vi "Init from Time Stamp.vi"(8 "error in":errorcluster, 10 "Time Stamp":timestamp format="%<%x %.3X>T", 11 "Time Stamp in":refnum<class "Time Stamp.lvclass">) -> (0 "error out":errorcluster, 3 "Time Stamp out":refnum<class "Time Stamp.lvclass">)   [LabVIEW 2023, in "HAL.lvlib" / "Time Stamp.lvclass"]
uses:
  Time Stamp.lvclass
  Time Stamp.lvclass/Time Stamp.ctl
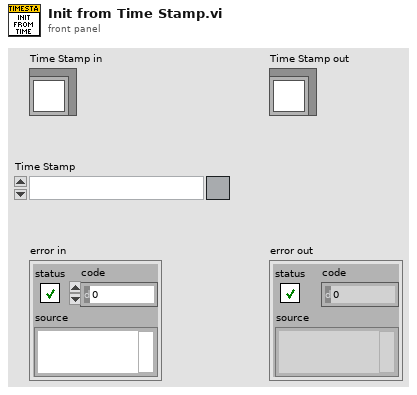
[diagram p1: front panel]
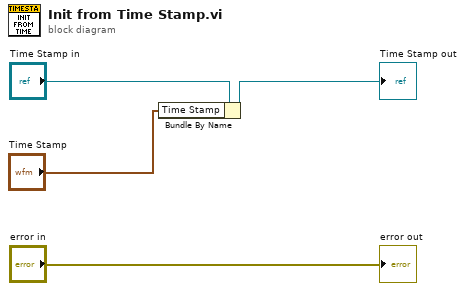
[diagram p0: block diagram]
diagram:
  n1 = Bundle By Name(cluster="Time Stamp in", "Time Stamp"="Time Stamp") -> (→"Time Stamp out":refnum<class "Time Stamp.lvclass">)
  "error out" <- "error in"
